vi "RUS_settings.vi"(0 "Lock-in DAQ settings":T3={"Lockin mode"=enum."NI-DAQ", "DAQmx Device"="Dev1", "SR Lockin"="GPIB0::10::INSTR", "Clock Multiplier"=64, "Low-pass filter"=enum."No filtering", "Ranges and couplings "=[{"Range"=1.0, "Coupling"=10106}], "Samples per read"=10, "Record IF"=FALSE, "Auto-phase"=FALSE, "RP IP Addres"="172.20.117.190"} {"Ranges and couplings"."Coupling" items=["default"=-1, "RSE"=10083, "NRSE"=10078, "Differential"=10106, "Pseudodifferential"=12529]}, 2 "Setup time, s/pt":dbl=5e-05, 5 "Save data settings":T1={"Save data"=TRUE, "Data Root Path"=path "", "File Prefix"="", "File Format"=enum."ASCII", "Save column names"=TRUE, "File Comments"="<Description of the current file>", "User/Prj"="<User Name/Project Description>"}, 9 "Fast swep settings":T7={"Update rate (Hz)"=250.0, "Start F, Hz"=200000.0, "Stop F"=250000.0, "Number of points"=50, "Amplitude"=2.1, "Init&amplitude"=TRUE, "IF"=1000.0, "Time constant"=0.01} {"IF" format="%#_6p"; "Amplitude" min=0.0 max=2.5; "Number of points" format="%.0p"; "Stop F" format="%#_6p"; "Start F, Hz" format="%#_6p"; "Update rate (Hz)" format="%0.2f"}, 13 "Output Representation":enum16{"Real/Imaginary", "Polar"}(ring)) -> (4 "RUS settings":T5={"NI-DAQ lockin settings"={"Samples per sine wave"=0, "Sine waves per freq step"=0, "Output Representation"=enum."Real/Imaginary", "Low-pass filter"=enum."Butterworth", "Ranges and couplings "=[]}, "Fast swep settings"={"Update rate (Hz)"=250.0, "Start F, Hz"=200000.0, "Stop F"=1700000.0, "Number of points"=30000, "Amplitude"=2.1, "Init&amplitude"=TRUE, "IF"=1000.0, "Time constant"=0.1}, "Pre-sweep delay, s"=0.0, "Lockin mode"=enum."NI-DAQ", "SR Lockin"="GPIB0::10::INSTR", "DAQmx Device"="Dev3", "Clock Multiplier"=64, "Fast Sweep Data Out"={"DO clock task"="", "DO task"="", "Update clock task"="", "DAQ lockin task"="", "Pre-sweep counter task"=""}, "Lockin Range, V"=0.0, "F Array"=[], "Freq. update clock terminal"="", "DO Clock Rate (Hz)"=5000000.0, "ADC clock terminal"="/PFI4", "Pre-sweep counter terminal"="", "Samples per read"=10, "DO clock terminal"="", "Pre-sweep points"=0, "F points per write"=1000, "Total sweep time, s"=0.0, "Initial SYNTH phase"=0.0, "Record IF"=FALSE, "Save data settings"={"Save data"=TRUE, "Data Root Path"=path "", "File Prefix"="", "File Format"=enum."ASCII", "Save column names"=TRUE, "File Comments"="<Description of the current file>", "User/Prj"="<User Name/Project Description>"}, "Data file path"=path "", "New data user event"=refnum, "Stop user event"=refnum, "Number of channels"=1, "Auto-phase"=FALSE, "RP Transeiver"=refnum} {"Lockin Range, V" format="%#_6e"; "Fast swep settings"."IF" format="%#_6p"; "Fast swep settings"."Amplitude" min=0.0 max=2.5; "Fast swep settings"."Number of points" format="%.0p"; "Fast swep settings"."Stop F" format="%#_6p"; "Fast swep settings"."Start F, Hz" format="%#_6p"; "Fast swep settings"."Update rate (Hz)" format="%0.2f"; "NI-DAQ lockin settings"."Ranges and couplings"."Coupling" items=["default"=-1, "RSE"=10083, "NRSE"=10078, "Differential"=10106, "Pseudodifferential"=12529]})   [LabVIEW 2018]
uses:
  resonant_ultrasound/Libraries/RUS/Controls/RUS settings.ctl
  NHMFL_Core/Libraries/Red Pitaya/RP Core/RP Transceiver/RP Transceiver.lvclass
  Users/arkady/Desktop/ado/github/NHMFL_Core/Libraries/Red Pitaya/RP Core/RP Instrument/RP Instrument.lvclass
  resonant_ultrasound/Libraries/RUS/Controls/RUS NI-DAQ Lockin Settings.ctl
  resonant_ultrasound/Libraries/RUS/Controls/Sweep settings.ctl
  resonant_ultrasound/Libraries/RUS/Controls/Lockin mode.ctl
  NHMFL_Core/Libraries/File/Controls/Save data settings.ctl
  NHMFL_Core/Libraries/File/Controls/File formats.ctl
  resonant_ultrasound/Libraries/RUS/Controls/Lock-in DAQ settings.ctl
  NHMFL_Core/Libraries/Red Pitaya/RP Core/RP Transceiver/Receiver format.ctl
  NHMFL_Core/Libraries/Red Pitaya/RP Core/RP Instrument/RP Instrument.lvclass/RP Instrument.ctl
  NHMFL_Core/Libraries/Red Pitaya/RP Core/RP Transceiver/RP Transceiver.lvclass/RP Transceiver.ctl
  NHMFL_Core/Libraries/Red Pitaya/RP Core/RP Instrument/Write Status check delay.vi
  NHMFL_Core/Libraries/Red Pitaya/RP Core/RP Transceiver/Write Receiver format.vi
  NHMFL_Core/Libraries/Red Pitaya/RP Core/RP Instrument/Write DDS delay.vi
  NHMFL_Core/Libraries/Red Pitaya/RP Core/RP Instrument/Write Server address.vi
panel:
  in  "RUS settings default":T5={"NI-DAQ lockin settings"={"Samples per sine wave"=0, "Sine waves per freq step"=0, "Output Representation"=enum."Real/Imaginary", "Low-pass filter"=enum."Butterworth", "Ranges and couplings "=[]}, "Fast swep settings"={"Update rate (Hz)"=250.0, "Start F, Hz"=200000.0, "Stop F"=1700000.0, "Number of points"=30000, "Amplitude"=2.1, "Init&amplitude"=TRUE, "IF"=1000.0, "Time constant"=0.1}, "Pre-sweep delay, s"=0.0, "Lockin mode"=enum."NI-DAQ", "SR Lockin"="GPIB0::10::INSTR", "DAQmx Device"="Dev3", "Clock Multiplier"=64, "Fast Sweep Data Out"={"DO clock task"="", "DO task"="", "Update clock task"="", "DAQ lockin task"="", "Pre-sweep counter task"=""}, "Lockin Range, V"=0.0, "F Array"=[], "Freq. update clock terminal"="", "DO Clock Rate (Hz)"=5000000.0, "ADC clock terminal"="PFI4", "Pre-sweep counter terminal"="", "Samples per read"=10, "DO clock terminal"="", "Pre-sweep points"=0, "F points per write"=1000, "Total sweep time, s"=0.0, "Initial SYNTH phase"=0.0, "Record IF"=FALSE, "Save data settings"={"Save data"=TRUE, "Data Root Path"=path "", "File Prefix"="", "File Format"=enum."ASCII", "Save column names"=TRUE, "File Comments"="<Description of the current file>", "User/Prj"="<User Name/Project Description>"}, "Data file path"=path "", "New data user event"=refnum, "Stop user event"=refnum, "Number of channels"=1, "Auto-phase"=FALSE, "RP Transeiver"=refnum} {"Lockin Range, V" format="%#_6e"; "Fast swep settings"."IF" format="%#_6p"; "Fast swep settings"."Amplitude" min=0.0 max=2.5; "Fast swep settings"."Number of points" format="%.0p"; "Fast swep settings"."Stop F" format="%#_6p"; "Fast swep settings"."Start F, Hz" format="%#_6p"; "Fast swep settings"."Update rate (Hz)" format="%0.2f"; "NI-DAQ lockin settings"."Ranges and couplings"."Coupling" items=["default"=-1, "RSE"=10083, "NRSE"=10078, "Differential"=10106, "Pseudodifferential"=12529]}
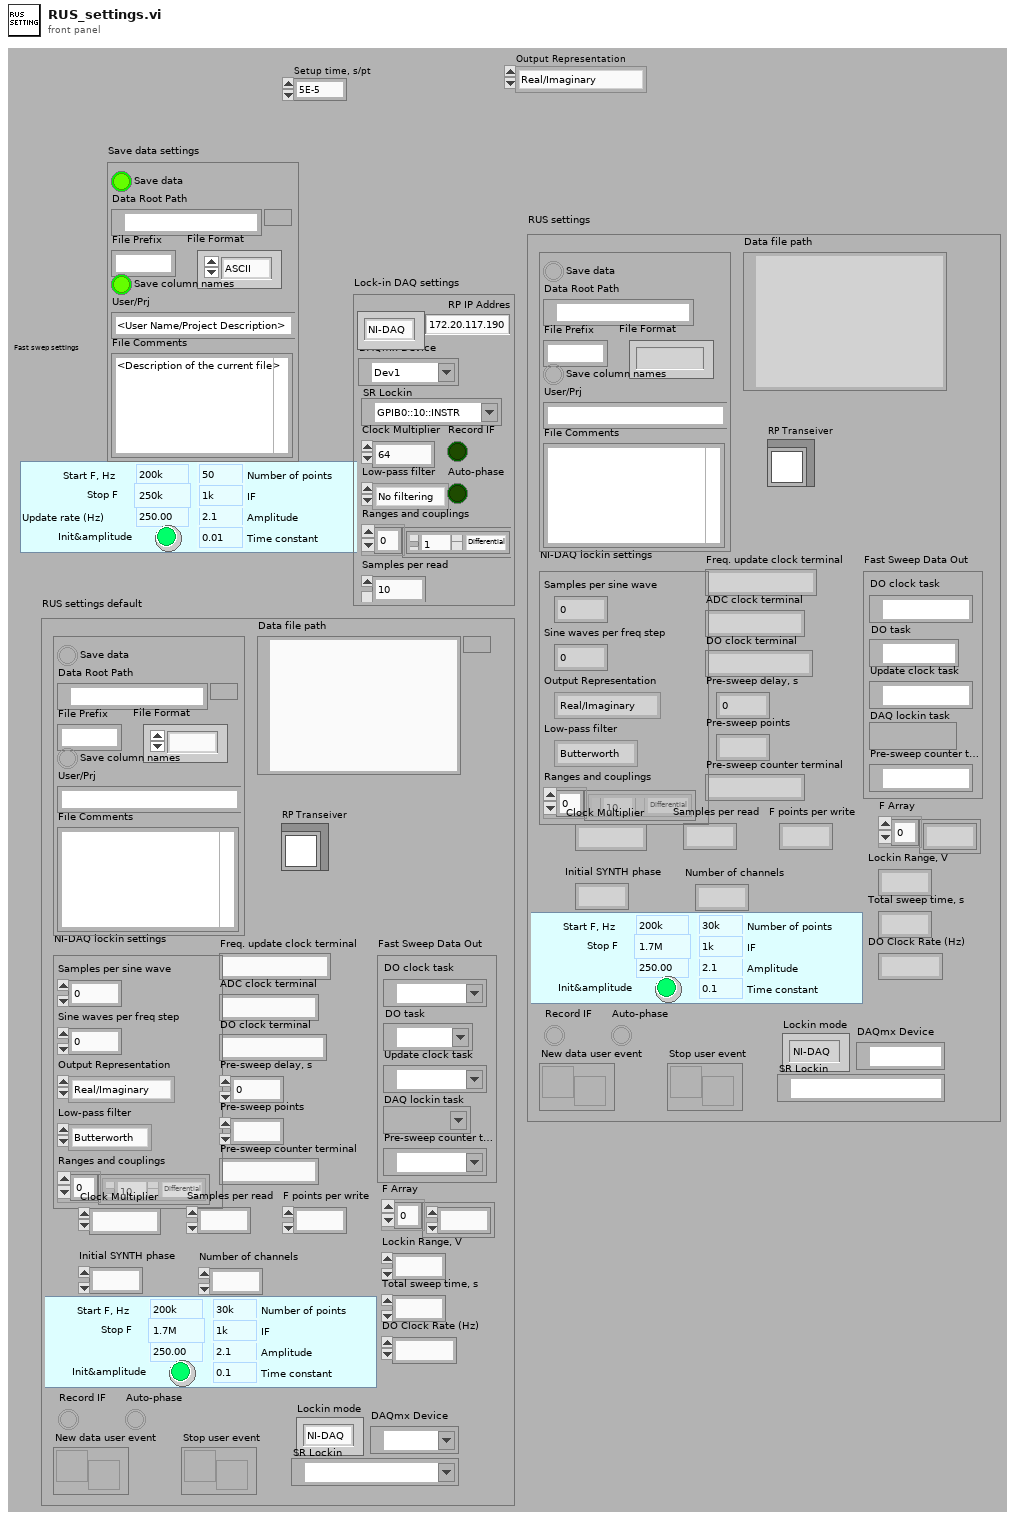
[diagram p1: front panel]
types:
  T1 = typedef "Save data settings.ctl" = cluster{"Save data":bool, "Data Root Path":path, "File Prefix":string, "File Format":T2, "Save column names":bool, "File Comments":string, "User/Prj":string}
  T2 = typedef "File formats.ctl" = enum16{"TDMS", "ASCII", "BINARY"}
  T3 = typedef "Lock-in DAQ settings.ctl" = cluster{"Lockin mode":T4, "DAQmx Device":tag, "SR Lockin":refnum<visa-resource-name>, "Clock Multiplier":i32, "Low-pass filter":enum16{"No filtering", "Butterworth", "Bessel"}, "Ranges and couplings ":cluster{"Range":dbl, "Coupling":i32}[], "Samples per read":i32, "Record IF":bool, "Auto-phase":bool, "RP IP Addres":string}
  T4 = typedef "Lockin mode.ctl" = enum16{"SRS", "NI-DAQ", "Pitaya"}
  T5 = typedef "RUS settings.ctl" = cluster{"NI-DAQ lockin settings":T6, "Fast swep settings":T7, "Pre-sweep delay, s":dbl, "Lockin mode":T4, "SR Lockin":refnum<visa-resource-name>, "DAQmx Device":tag, "Clock Multiplier":i32, "Fast Sweep Data Out":cluster{"DO clock task":refnum<k21>, "DO task":refnum<k21>, "Update clock task":refnum<k21>, "DAQ lockin task":refnum<k21>, "Pre-sweep counter task":refnum<k21>}, "Lockin Range, V":sgl, "F Array":dbl[], "Freq. update clock terminal":string, "DO Clock Rate (Hz)":dbl, "ADC clock terminal":string, "Pre-sweep counter terminal":string, "Samples per read":i32, "DO clock terminal":string, "Pre-sweep points":i32, "F points per write":i32, "Total sweep time, s":dbl, "Initial SYNTH phase":dbl, "Record IF":bool, "Save data settings":T1, "Data file path":path, "New data user event":refnum<user-event>, "Stop user event":refnum<user-event>, "Number of channels":i32, "Auto-phase":bool, "RP Transeiver":refnum<class "RP Transceiver.lvclass">}
  T6 = typedef "RUS NI-DAQ Lockin Settings.ctl" = cluster{"Samples per sine wave":i32, "Sine waves per freq step":i32, "Output Representation":enum16{"Real/Imaginary", "Polar"}, "Low-pass filter":enum16{"No filtering", "Butterworth", "Bessel"}, "Ranges and couplings ":cluster{"Range":dbl, "Coupling":i32}[]}
  T7 = typedef "Sweep settings.ctl" = cluster{"Update rate (Hz)":dbl, "Start F, Hz":dbl, "Stop F":dbl, "Number of points":i32, "Amplitude":dbl, "Init&amplitude":bool, "IF":dbl, "Time constant":dbl}
  T8 = typedef "Receiver format.ctl" = enum16{"X-Y-F", "F-X-Y", "X-Y", "X"}
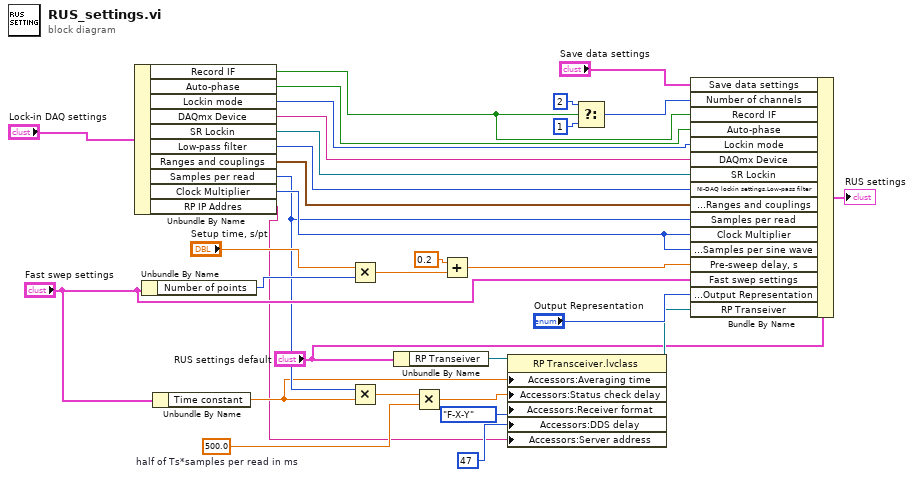
[diagram p0: block diagram]
diagram:
  w5 = 500.0  # half of Ts*samples per read in ms
  n1 = Unbundle By Name("Lock-in DAQ settings") -> ("Record IF"=w16:bool, "Auto-phase"=w14:bool, "Lockin mode"=w25:T4, "DAQmx Device"=w24:tag, "SR Lockin"=w23:refnum<visa-resource-name>, "Low-pass filter"=w21:enum16{"No filtering", "Butterworth", "Bessel"}, "Ranges and couplings"=w20:cluster{"Range":dbl, "Coupling":i32}[], "Samples per read"=w8:i32, "Clock Multiplier"=w22:i32, "RP IP Addres"=w1:string)
  n2 = Unbundle By Name("Fast swep settings") -> ("Number of points"=w30:i32)
  n3 = Unbundle By Name("Fast swep settings") -> ("Time constant"=w7:dbl)
  n4 = Multiply(x="Setup time, s/pt", y=w30) -> (x*y=w28:dbl)
  n5 = Multiply(x=w8, y=w7) -> (x*y=w6:dbl)
  n6 = Unbundle By Name("RUS settings default") -> ("RP Transeiver"=w9:refnum<class "RP Transceiver.lvclass">)
  n7 = Multiply(x=w6, y=w5) -> (x*y=w4:dbl)
  n8 = Add(x=0.2, y=w28) -> (x+y=w29:dbl)
  n9 = property class="RP Transceiver.lvclass"(reference=w9, "Accessors:Averaging time"=w7, "Accessors:Status check delay"=w4, "Accessors:Receiver format"=Receiver_format."F-X-Y" ("Receiver format"), "Accessors:DDS delay"=u32 47 ("DDS delay"), "Accessors:Server address"=w1) -> (reference out=w13:refnum<class "RP Transceiver.lvclass">)  [unwired: 1 in, 1 out]
  n10 = Select(t=2 ("Number of channels"), s=w16, f=1) -> (s? t:f=w15:i32)
  n11 = Bundle By Name(cluster="RUS settings default", "Save data settings"="Save data settings", "Number of channels"=w15, "Record IF"=w16, "Auto-phase"=w14, "Lockin mode"=w25, "DAQmx Device"=w24, "SR Lockin"=w23, "NI-DAQ lockin settings.Low-pass filter"=w21, "NI-DAQ lockin settings.Ranges and couplings"=w20, "Samples per read"=w8, "Clock Multiplier"=w22, "NI-DAQ lockin settings.Samples per sine wave"=w22, "Pre-sweep delay, s"=w29, "Fast swep settings"="Fast swep settings", "NI-DAQ lockin settings.Output Representation"="Output Representation", "RP Transeiver"=w13) -> (→"RUS settings":T5)
